vi "CAN.Cleanup.vi"(8 "error in (no error)":errorcluster, 11 "State Variables Out":T1={"Comm"=refnum, "Parameters"={"Name"="", "CAN"={"Interface"="", "Baud Rate"=0, "Diagnostic Protocol"=enum."GMLAN", "Transport Protocol"=enum."ISO TP - Normal Mode", "Transmit ID"=0, "Receive ID"=0, "Transmit Extension"=0, "Receive Extension"=0, "Receive UUDT ID"=0, "Enable Stream"=FALSE, "VW TP Channel ID"=0, "Fill Frame"=FALSE, "Fill Byte"=0, "Termination"=FALSE, "LIN Cluster"="", "NAD"=0, "IO Mode"=0, "Max DLC"=0, "FD Baud Rate"=0, "Timeout"=0, "FD ISO Mode"=0, "DoIP Address"="", "DoIP Source Address"=3584, "DoIP Dynamic Port"=TRUE, "DoIP Version"=2}, "986x"={"Enable"=FALSE, "RIO Device"="", "Bitfile"=path ""}, "Reads"=[], "Frames Lookup"=variant, "Writes"=[], "DPIDs"=[], "DPID Lookup"=variant, "DTC"={"Descriptor"={"DTC Byte Length"=0, "Status Byte Length"=0, "Add Data Byte Length"=0, "Byte Order"=enum."Motorola"}, "Value.Code"=[], "Value.String"=[], "Value.J2012String"=[], "Status.Code"=[], "Status.String"=[]}, "Created DTCs"=0, "Polls"=[], "Service Channels Status Lookup"=variant, "Trigger Lookup"=variant, "Security"={"Type"=enum."None", "Source DLL Path"=path "", "Target DLL Path"=path "", "Security Level"=0, "Static Master Key"="", "Max Key Length"=1, "Host IP Address"=""}, "Initial Comm State"=FALSE}, "ADCS Connection"={"Diag CAN Handle"=0, "Transport Protocol"=enum."ISO TP - Normal Mode", "Receive Address Extension"=0, "Transmit Address Extension"=0, "Receive CAN Id"=0, "Transmit CAN Id"=0, "Log Frames ?"=FALSE, "My TP Address"=0, "Other TP Address"=0, "T1"=0, "T2"=0, "T3"=0, "T4"=0, "Tx SN"=0, "Block Size"=0, "Rx SN"=0, "VW TP Initialized?"=FALSE, "Tx block no"=0, "baud rate"=0, "Interface"="", "Channel Diag CAN Handle"=0, "UDP Connection ID"=refnum, "TCP Connection ID"=refnum, "Target IP Addr"=0, "Source Address"=0, "Target Address"=0, "Send Header NACK?"=FALSE, "DLL Handle"=0, "NAD"=0, "Time Stamp read first"=0.0, "Time Stamp read last"=0.0, "Time Stamp write first"=0.0, "Time Stamp write last"=0.0, "Time Stamp write"=0.0, "Time Stamp read"=0.0, " I/O Mode"=0, "FD Baudrate"=0, "TX_DL"=0, "RX_DL"=0, "DoIP Protocol Version"=0, " Selected I/O Mode"=0, "TesterPresent Counter"=0, "TesterPresent Limit"=0, "TesterPresent Tick[ms]"=0, "TesterPresent RequireResponse?"=FALSE, "TesterPresent Stored Ref?"=FALSE, "TesterPresent Message"=[], "TesterPresent Task Handle"=0, "TesterPresent Semaphore"=refnum, "Response Plausibility Check"=0, "Default Version?"=FALSE, "Diagostic Globals"={"Timeout FC (Bs)"=0, "Timeout CF (Cr)"=0, "Timeout Diag Command"=0, "Receive Block Size (BS)"=0, "Wait Time CF (STmin)"=0, "Max Waits (N_WFTmax)"=0, "Waits to Send (N_WAIT)"=0, "Time between Waits (TW)"=0, "Fill CAN Frames?"=FALSE, "Fill Byte"=0, "Invalid Response as Error?"=FALSE, "Max RspPending Count"=0, "VWTP Command Timeout"=0, "Transport Protocol"=enum."ISO TP - Normal Mode", "Diag CAN Handle"=0, "DLL Handle"=0, "Timeout RspPending"=0}, "Session-based Properties?"=FALSE}, "XNET References"={"Database"="", "GMLAN.DPID.Frame"="", "Cluster.Convert"=""}, "XNETEngine (GMLAN)"=refnum, "Process"=refnum, "Reads"=refnum, "Writes"=refnum, "Cmds"=refnum, "DTCs"=refnum, "DTC Count"=refnum, "Status"=refnum, "Triggers"=refnum, "CANConnected"=refnum, "LocalStop"=refnum, "LocalCommStatus"=refnum, "Service Channels Status"=refnum, "Settings"=refnum, "Streaming Refs"={"Addon"="", "Port"="", "Filter Ref"=refnum, "Default Filter"={"ID Filters"=[], "Direction Filter"=enum."Tx/Rx", "Type Filter"=enum."All"}, "Port Settings"={"Mode"=0, "Baud Rate"=0, "Termination"=0, "FD ISO Mode"=0, "FD Baud Rate"=0}}} {"Streaming Refs"."Port Settings"."FD ISO Mode" items=["ISO", "Non ISO", "ISO Legacy"]; "Streaming Refs"."Port Settings"."Termination" items=["Off", "On"]; "Streaming Refs"."Port Settings"."Mode" items=["CAN 2.0", "CAN FD", "CAN FD+BRS"]; "ADCS Connection"."Diagostic Globals"."Fill Byte" format="%x"; "ADCS Connection"."TesterPresent Message" format="%.0x"; "ADCS Connection"."Selected I/O Mode" items=["CAN", "CAN FD", "CAN FD+BRS", "ECU Determined"]; "ADCS Connection"."DoIP Protocol Version" items=["2010"=1, "2012"=2]; "ADCS Connection"."RX_DL" items=["8"=8, "12"=12, "16"=16, "20"=20, "24"=24, "32"=32, "48"=48, "64"=64]; "ADCS Connection"."TX_DL" items=["8"=8, "12"=12, "16"=16, "20"=20, "24"=24, "32"=32, "48"=48, "64"=64]; "ADCS Connection"."I/O Mode" items=["CAN", "CAN FD", "CAN FD+BRS", "Not yet determined"]; "Parameters"."Writes"."Signals"."Byte Order" items=["Little Endian", "Big Endian"]; "Parameters"."Writes"."Signals"."Data Type" items=["Signed", "Unsigned", "IEEE Float"]; "Parameters"."CAN"."DoIP Version" items=["2010"=1, "2012"=2]; "Parameters"."CAN"."DoIP Source Address" format="%.0x"; "Parameters"."CAN"."FD ISO Mode" items=["ISO", "Non ISO", "ISO Legacy"]; "Parameters"."CAN"."IO Mode" items=["CAN 2.0", "CAN FD", "CAN FD+BRS"]; "Parameters"."CAN"."Fill Byte" format="%.0x"; "Parameters"."CAN"."VW TP Channel ID" format="%.0x"; "Parameters"."CAN"."Receive UUDT ID" format="%.0x"; "Parameters"."CAN"."Receive Extension" format="%.0x"; "Parameters"."CAN"."Transmit Extension" format="%.0x"; "Parameters"."CAN"."Receive ID" format="%.0x"; "Parameters"."CAN"."Transmit ID" format="%.0x"; "Parameters"."Reads"."Signals"."Byte Order" items=["Little Endian", "Big Endian"]; "Parameters"."Reads"."Signals"."Data Type" items=["Signed", "Unsigned", "IEEE Float"]}) -> (0 "error out":errorcluster)   [LabVIEW 2019, in "Diagnostics Addon Engine.lvlib"]
uses:
  Diagnostics Addon Engine.lvlib
  Types/Diagnostics.State.ctl
  <vilib>/NI/NI VeriStand Addon Network Comm/Engine/VeriStand Comm.lvclass
  <vilib>/NI/NIVS Inline Async API/_VS Inline Async API/Process/Process.lvclass
  Addon Shared/Types/SysDef.Compile.ctl
  Addon Shared/Types/CAN.ctl
  Addon Shared/Types/CAN.Interface.ctl
  Addon Shared/Types/Protocol.ctl
  Addon Shared/Types/Transport.ctl
  Addon Shared/Types/986x.ctl
  Addon Shared/Types/Frame.Compile.ctl
  Addon Shared/Types/Type.ctl
  Addon Shared/Types/Signal.ctl
  Addon Shared/Types/DPID.ctl
  Addon Shared/Types/DPID.Rate.ctl
  Addon Shared/Types/DTC.Settings.ctl
  Addon Shared/Types/DTC.Descriptor.ctl
  Addon Shared/Types/Poll.Compiled.ctl
  Addon Shared/Types/Security.ctl
  Addon Shared/Types/Security.Type.ctl
  <vilib>/Automotive Diagnostic Command Set/Diagnostic Transport.llb/Diag Reference.ctl
  <vilib>/Automotive Diagnostic Command Set/Diagnostic Transport.llb/Transport Protocol Selector.ctl
  <vilib>/Automotive Diagnostic Command Set/Diagnostic Transport.llb/DoIP Protocol Version.ctl
  <vilib>/Automotive Diagnostic Command Set/Diagnostic Transport.llb/Diag Globals.ctl
  Types/XNET.Refs.ctl
  <vilib>/NI/AMC/Message Queue.ctl
  <vilib>/NI/AMC/Message.ctl
  <vilib>/NI/Tools/Keyed Array/KeyedArray.ctl
  <vilib>/NI/NIVS Inline Async API/_Data Access Engine/Data Access Engine/Types/Write.DVR.ctl
  <vilib>/NI/NIVS Inline Async API/_Data Access Engine/Access Type Classes/Write/Write.lvclass
  <vilib>/NI/NIVS Inline Async API/_Data Access Engine/Data Access Engine/Types/Read.DVR.ctl
  <vilib>/NI/NIVS Inline Async API/_Data Access Engine/Access Type Classes/Read/Read.lvclass
  <vilib>/NI/NIVS Inline Async API/_Data Access Engine/Data Access Engine/Types/ReadWrite.DVR.ctl
  <vilib>/NI/NIVS Inline Async API/_Data Access Engine/Access Type Classes/ReadWrite/ReadWrite.lvclass
  SubModules/CAN-Streaming-Support/Source/Addon/Addon Engine/Types/Engine Stream Refs.ctl
  SubModules/CAN-Streaming-Support/Source/Addon/Addon Shared/Types/Direction Filter.ctl
  SubModules/CAN-Streaming-Support/Source/Addon/Addon Shared/Types/Type Filter.ctl
  SubModules/CAN-Streaming-Support/Source/Addon/Addon Shared/Types/Filter Parameters.ctl
  SubModules/CAN-Streaming-Support/Source/Addon/Addon Engine/Types/Engine Stream Port Settings.ctl
  <vilib>/NI/NIVS Inline Async API/_Data Access Engine/Access Type Classes/Write/Write.lvclass/Write.ctl
  <vilib>/NI/NIVS Inline Async API/_Data Access Engine/Data Access Engine/Methods/Write.Data.vi
  <vilib>/NI/NIVS Inline Async API/_Data Access Engine/Access Type Classes/Write/Write.ProcessData.vi
  <vilib>/NI/NIVS Inline Async API/_Data Access Engine/Access Type Classes/Write/Write.Buffer.vi
  <vilib>/NI/NIVS Inline Async API/_Data Access Engine/Access Type Classes/Write/Write.Commit.vi
  Addon Shared/SubVIs/Constants.vi
  <vilib>/xnet/xnet.llb/XNET Database Delete (Cluster).vi
  <vilib>/xnet/xnet.llb/XNET Database Close (Database).vi
  <vilib>/Utility/SystemLogging/Write to System Log.vi
  <vilib>/addons/Automotive Diagnostic Command Set/NI_Automotive Diagnostic Command Set.lvlib
  <vilib>/NI/NIVS Inline Async API/_Data Access Engine/Data Access Engine/Data Access Engine.lvclass
  Addon Shared/Diagnostics Addon Shared.lvlib
  <vilib>/NI/Tools/Keyed Array/Tools_KeyedArray.lvlib
  <vilib>/NI/AMC/AMC.lvlib
  SubModules/CAN-Streaming-Support/Source/Addon/Addon Engine/CAN Stream Support Engine.lvlib
  SubModules/CAN-Streaming-Support/Source/Addon/Addon Shared/CAN Stream Support Shared.lvlib
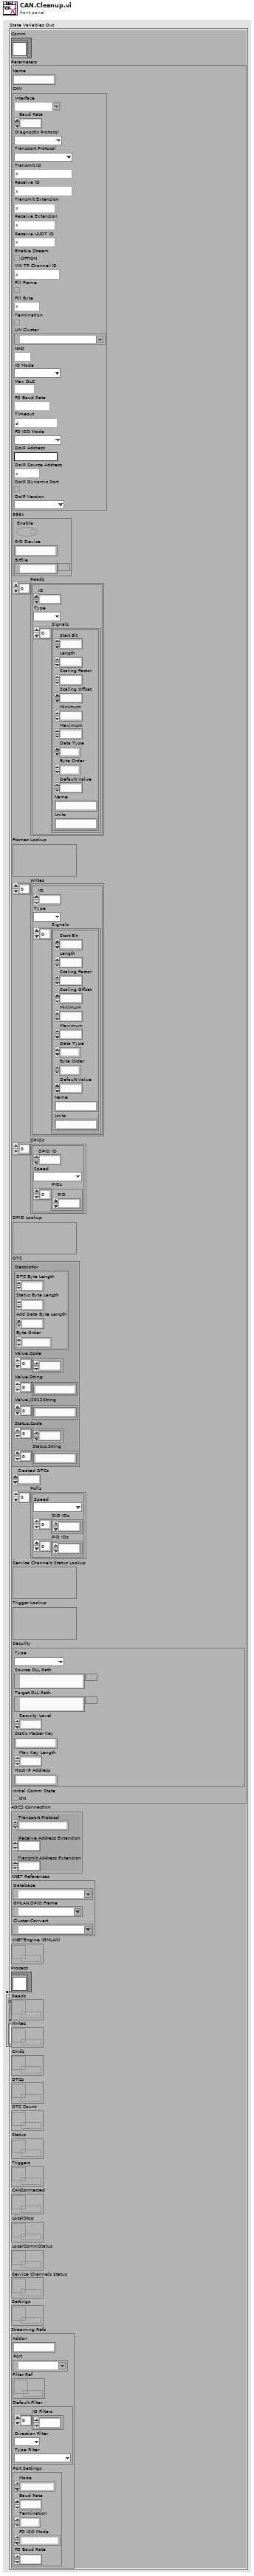
[diagram p1: front panel]
types:
  T1 = typedef "Diagnostics Addon Engine.lvlib/Diagnostics.State.ctl" = cluster{"Comm":refnum<class "VeriStand Comm.lvclass">, "Parameters":T2, "ADCS Connection":T18, "XNET References":T23, "XNETEngine (GMLAN)":T24, "Process":refnum<class "Process.lvclass">, "Reads":T25, "Writes":T26, "Cmds":T27, "DTCs":T25, "DTC Count":T25, "Status":T25, "Triggers":T27, "CANConnected":T25, "LocalStop":refnum<data-value>, "LocalCommStatus":refnum<data-value>, "Service Channels Status":T25, "Settings":T26, "Streaming Refs":T28}
  T2 = typedef "Diagnostics Addon Shared.lvlib/SysDef.Compile.ctl" = cluster{"Name":string, "CAN":T3, "986x":T7, "Reads":T8[], "Frames Lookup":variant, "Writes":T8[], "DPIDs":T11[], "DPID Lookup":variant, "DTC":T13, "Created DTCs":u32, "Polls":T15[], "Service Channels Status Lookup":variant, "Trigger Lookup":variant, "Security":T16, "Initial Comm State":bool}
  T3 = typedef "Diagnostics Addon Shared.lvlib/CAN.ctl" = cluster{"Interface":T4, "Baud Rate":u64, "Diagnostic Protocol":T5, "Transport Protocol":T6, "Transmit ID":u32, "Receive ID":u32, "Transmit Extension":u8, "Receive Extension":u8, "Receive UUDT ID":u32, "Enable Stream":bool, "VW TP Channel ID":u32, "Fill Frame":bool, "Fill Byte":u8, "Termination":bool, "LIN Cluster":refnum<k21>, "NAD":u8, "IO Mode":u32, "Max DLC":u16, "FD Baud Rate":u64, "Timeout":u32, "FD ISO Mode":u32, "DoIP Address":string, "DoIP Source Address":u16, "DoIP Dynamic Port":bool, "DoIP Version":u16}
  T4 = typedef "Diagnostics Addon Shared.lvlib/CAN.Interface.ctl" = string
  T5 = typedef "Diagnostics Addon Shared.lvlib/Protocol.ctl" = enum16{"GMLAN", "KWP-2000", "UDS", "User-Defined"}
  T6 = typedef "Diagnostics Addon Shared.lvlib/Transport.ctl" = enum16{"ISO TP - Normal Mode", "ISO TP - Mixed Mode", "VW TP 2.0", "Diagnostics on IP", "ISO TP LIN"}
  T7 = typedef "Diagnostics Addon Shared.lvlib/986x.ctl" = cluster{"Enable":bool, "RIO Device":string, "Bitfile":path}
  T8 = typedef "Diagnostics Addon Shared.lvlib/Frame.Compile.ctl" = cluster{"ID":u32, "Type":T9, "Signals":T10[]}
  T9 = typedef "Diagnostics Addon Shared.lvlib/Type.ctl" = enum16{"DID", "CDID", "PID", "CPID", "Read Memory", "Write Memory", "IO Control", "Routine Start", "Routine Request", "Routine Stop", "User Defined", "DTC Control", "Clear DTCs", "Read DTCs", "Start DTCs", "DTC Change Count", "Tester Present", "Unlock ECU", "Reset ECU", "Diag Session Control", "Communication Control", "DPID Control", "Poll Control", "Diag Comm Port Control"}
  T10 = typedef "Diagnostics Addon Shared.lvlib/Signal.ctl" = cluster{"Start Bit":u32, "Length":u32, "Scaling Factor":dbl, "Scaling Offset":dbl, "Minimum":dbl, "Maximum":dbl, "Data Type":u32, "Byte Order":u32, "Default Value":dbl, "Name":string, "Units":string}
  T11 = typedef "Diagnostics Addon Shared.lvlib/DPID.ctl" = cluster{"DPID ID":u8, "Speed":T12, "PIDs":u16[]}
  T12 = typedef "Diagnostics Addon Shared.lvlib/DPID.Rate.ctl" = enum16{"Slow", "Medium", "Fast"}
  T13 = typedef "Diagnostics Addon Shared.lvlib/DTC.Settings.ctl" = cluster{"Descriptor":T14, "Value.Code":dbl[], "Value.String":string[], "Value.J2012String":string[], "Status.Code":dbl[], "Status.String":string[]}
  T14 = typedef "Diagnostics Addon Shared.lvlib/DTC.Descriptor.ctl" = cluster{"DTC Byte Length":i32, "Status Byte Length":i32, "Add Data Byte Length":i32, "Byte Order":enum16{"Motorola", "Intel"}}
  T15 = typedef "Diagnostics Addon Shared.lvlib/Poll.Compiled.ctl" = cluster{"Speed":T12, "DID IDs":u32[], "PID IDs":u32[]}
  T16 = typedef "Diagnostics Addon Shared.lvlib/Security.ctl" = cluster{"Type":T17, "Source DLL Path":path, "Target DLL Path":path, "Security Level":u8, "Static Master Key":string, "Max Key Length":u32, "Host IP Address":string}
  T17 = typedef "Diagnostics Addon Shared.lvlib/Security.Type.ctl" = enum16{"None", "SeedKey DLL", "MasterKey (Channel)", "MasterKey (Static)", "SeedKey DLL (Windows)"}
  T18 = typedef "NI_Automotive Diagnostic Command Set.lvlib/Diag Reference.ctl" = cluster{"Diag CAN Handle":u32, "Transport Protocol":T19, "Receive Address Extension":u8, "Transmit Address Extension":u8, "Receive CAN Id":u32, "Transmit CAN Id":u32, "Log Frames ?":bool, "My TP Address":u8, "Other TP Address":u8, "T1":u16, "T2":u16, "T3":u16, "T4":u16, "Tx SN":u8, "Block Size":u8, "Rx SN":u8, "VW TP Initialized?":bool, "Tx block no":u8, "baud rate":u64, "Interface":string, "Channel Diag CAN Handle":u32, "UDP Connection ID":refnum<k16>, "TCP Connection ID":refnum<k5>, "Target IP Addr":u32, "Source Address":u16, "Target Address":u16, "Send Header NACK?":bool, "DLL Handle":u32, "NAD":u8, "Time Stamp read first":dbl, "Time Stamp read last":dbl, "Time Stamp write first":dbl, "Time Stamp write last":dbl, "Time Stamp write":dbl, "Time Stamp read":dbl, " I/O Mode":u32, "FD Baudrate":u64, "TX_DL":u16, "RX_DL":u16, "DoIP Protocol Version":T20, " Selected I/O Mode":u32, "TesterPresent Counter":u32, "TesterPresent Limit":u32, "TesterPresent Tick[ms]":i32, "TesterPresent RequireResponse?":bool, "TesterPresent Stored Ref?":bool, "TesterPresent Message":u8[], "TesterPresent Task Handle":i32, "TesterPresent Semaphore":T21, "Response Plausibility Check":u32, "Default Version?":bool, "Diagostic Globals":T22, "Session-based Properties?":bool}
  T19 = typedef "NI_Automotive Diagnostic Command Set.lvlib/Transport Protocol Selector.ctl" = enum16{"ISO TP - Normal Mode", "ISO TP - Mixed Mode", "VW TP 2.0", "Diagnostics on IP", "ISO TP LIN"}
  T20 = typedef "NI_Automotive Diagnostic Command Set.lvlib/DoIP Protocol Version.ctl" = u8
  T21 = typedef "Semaphore RefNum" = refnum<k1>
  T22 = typedef "NI_Automotive Diagnostic Command Set.lvlib/Diag Globals.ctl" = cluster{"Timeout FC (Bs)":u32, "Timeout CF (Cr)":u32, "Timeout Diag Command":u32, "Receive Block Size (BS)":u8, "Wait Time CF (STmin)":u8, "Max Waits (N_WFTmax)":u8, "Waits to Send (N_WAIT)":i32, "Time between Waits (TW)":u32, "Fill CAN Frames?":bool, "Fill Byte":u32, "Invalid Response as Error?":bool, "Max RspPending Count":u32, "VWTP Command Timeout":u32, "Transport Protocol":T19, "Diag CAN Handle":u32, "DLL Handle":u32, "Timeout RspPending":u32}
  T23 = typedef "Diagnostics Addon Engine.lvlib/XNET.Refs.ctl" = cluster{"Database":refnum<k21>, "GMLAN.DPID.Frame":refnum<k21>, "Cluster.Convert":refnum<k21>}
  T24 = typedef "AMC.lvlib/Message Queue.ctl" = refnum<queue>
  T25 = typedef "Data Access Engine.lvlib/Data Access Engine.lvclass/Write.DVR.ctl" = refnum<data-value>
  T26 = typedef "Data Access Engine.lvlib/Data Access Engine.lvclass/Read.DVR.ctl" = refnum<data-value>
  T27 = typedef "Data Access Engine.lvlib/Data Access Engine.lvclass/ReadWrite.DVR.ctl" = refnum<data-value>
  T28 = typedef "CAN Stream Support Engine.lvlib/Engine Stream Refs.ctl" = cluster{"Addon":string, "Port":refnum<k21>, "Filter Ref":refnum<data-value>, "Default Filter":T29, "Port Settings":T32}
  T29 = typedef "CAN Stream Support Shared.lvlib/Filter Parameters.ctl" = cluster{"ID Filters":u32[], "Direction Filter":T30, "Type Filter":T31}
  T30 = typedef "CAN Stream Support Shared.lvlib/Direction Filter.ctl" = enum16{"Tx/Rx", "Rx", "Tx"}
  T31 = typedef "CAN Stream Support Shared.lvlib/Type Filter.ctl" = enum16{"All", "CAN Data", "CAN Remote", "CAN Bus Error", "CAN 2.0 Data", "CAN FD Data", "CAN FD+BRS Data", "J1939 Data", "Delay", "Log Trigger", "Start Trigger"}
  T32 = typedef "CAN Stream Support Engine.lvlib/Engine Stream Port Settings.ctl" = cluster{"Mode":u32, "Baud Rate":u64, "Termination":u32, "FD ISO Mode":u32, "FD Baud Rate":u64}
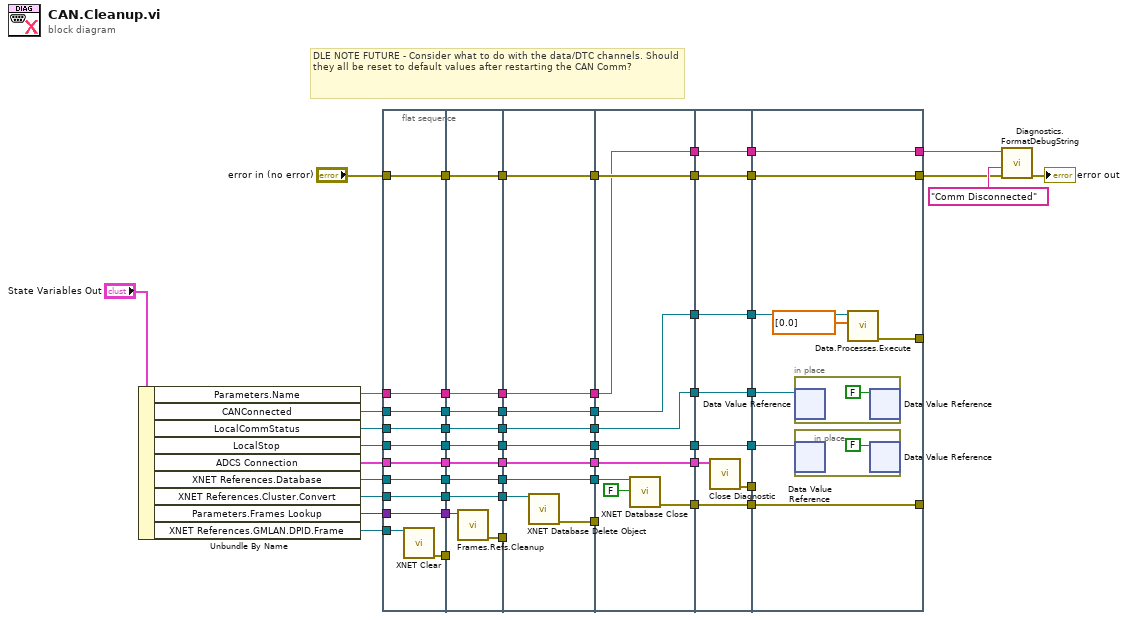
[diagram p0: block diagram]
diagram:
  # "DLE NOTE FUTURE - Consider what to do with the data/DTC channels. Should they all be reset to default values after restarting the CAN Comm?"
  n1 = Unbundle By Name("State Variables Out") -> ("Parameters.Name"=w13:string, "CANConnected"=w26:T25, "LocalCommStatus"=w27:refnum<data-value>, "LocalStop"=w25:refnum<data-value>, "ADCS Connection"=w22:T18, "XNET References.Database"=w21:refnum<k21>, "XNET References.Cluster.Convert"=w20:refnum<k21>, "Parameters.Frames Lookup"=w19:variant, "XNET References.GMLAN.DPID.Frame"=w18:refnum<k21>)
  n2 = flat-sequence {
    tunnel: w20 -> [w66]
    tunnel: w19 -> [w67]
    tunnel: [w67] -> w56
    tunnel: [w66] -> w55
    tunnel: w18 -> [w65]
    tunnel: [w64] -> w54
    tunnel: [w63] -> w53
    tunnel: w22 -> [w63]
    tunnel: [w62] -> w52
    tunnel: w21 -> [w62]
    tunnel: "error in (no error)" -> [w61]
    tunnel: [w61] -> w51
    tunnel: [w60] -> w50
    tunnel: w25 -> [w60]
    tunnel: [w59] -> w49
    tunnel: w26 -> [w59]
    tunnel: w27 -> [w58]
    tunnel: [w58] -> w48
    tunnel: [w57] -> w14
    tunnel: w13 -> [w57]
    tunnel: [w77] -> w47
    tunnel: w56 -> [w76]
    tunnel: w55 -> [w77]
    tunnel: w54 -> [_]
    tunnel: [w75] -> w46
    tunnel: w53 -> [w75]
    tunnel: [w74] -> w45
    tunnel: w52 -> [w74]
    tunnel: [w73] -> w44
    tunnel: [w72] -> w43
    tunnel: w51 -> [w72]
    tunnel: [w71] -> w42
    tunnel: w50 -> [w71]
    tunnel: [w70] -> w41
    tunnel: w49 -> [w70]
    tunnel: [w69] -> w40
    tunnel: w48 -> [w69]
    tunnel: [w68] -> w15
    tunnel: w14 -> [w68]
    tunnel: [w86] -> w8
    tunnel: [w85] -> w7
    tunnel: [w84] -> w6
    tunnel: [w83] -> w5
    tunnel: [w82] -> w4
    tunnel: [w81] -> w3
    tunnel: [w80] -> w2
    tunnel: w15 -> [w80]
    tunnel: w40 -> [w81]
    tunnel: w41 -> [w82]
    tunnel: w42 -> [w83]
    tunnel: w43 -> [w84]
    tunnel: w44 -> [_]
    tunnel: w45 -> [w85]
    tunnel: w46 -> [w86]
    tunnel: w47 -> [w79]
    tunnel: [w78] -> w1
    tunnel: [w93] -> w39
    tunnel: w8 -> [w95]
    tunnel: [w95] -> w38
    tunnel: w7 -> [w94]
    tunnel: [w91] -> w37
    tunnel: w6 -> [w91]
    tunnel: [w90] -> w36
    tunnel: w5 -> [w90]
    tunnel: [w89] -> w35
    tunnel: w4 -> [w89]
    tunnel: [w88] -> w34
    tunnel: w3 -> [w88]
    tunnel: [w87] -> w16
    tunnel: w2 -> [w87]
    tunnel: w1 -> [_]
    tunnel: w39 -> [w103]
    tunnel: w38 -> [w102]
    tunnel: w37 -> [w101]
    tunnel: [w103] -> w33
    tunnel: [w101] -> w32
    tunnel: [w100] -> w31
    tunnel: [w99] -> w30
    tunnel: w36 -> [w99]
    tunnel: w35 -> [w98]
    tunnel: [w98] -> w29
    tunnel: [w97] -> w28
    tunnel: w34 -> [w97]
    tunnel: [w96] -> w17
    tunnel: w16 -> [w96]
    tunnel: [w110] -> w10
    tunnel: [w111] -> _
    tunnel: w33 -> [w111]
    tunnel: w32 -> [w110]
    tunnel: w31 -> [_]
    tunnel: w30 -> [w109]
    tunnel: w29 -> [w107]
    tunnel: [w106] -> _
    tunnel: w28 -> [w105]
    tunnel: w17 -> [w104]
    tunnel: [w104] -> w11
    frame #0 {
      n3 = call <vilib>:"XNET Clear.vi"("session in"=w65) -> ("error out"=w64:errorcluster)  [unwired: 14 in]
    }
    frame #1 {
      n4 = call "Frames.Refs.Cleanup.vi"("Lookup"=w76) -> ("Array"=w73:errorcluster[])  [unwired: 10 in]
    }
    frame #2 {
      n5 = call-poly <vilib>:"XNET Database Delete Object.vi"("cluster in"=w79) -> ("error out"=w78:errorcluster)  [unwired: 14 in]
    }
    frame #3 {
      n6 = call-poly <vilib>:"XNET Database Close.vi"("database in"=w94, "close all? (true)"=FALSE) -> ("error out"=w93:errorcluster)  [unwired: 13 in]
    }
    frame #4 {
      n7 = call <vilib>:"Close Diagnostic.vi"("diag ref in"=w102) -> ("error out"=w100:errorcluster)  [unwired: 10 in]
    }
    frame #5 {
      n8 = in-place {
        n9 = in-place-dvr #1(w105) -> ()  [unwired: 2 out]
        n10 = in-place-dvr #1(FALSE ("data value")) -> ()  [unwired: 2 out]
      }
      n11 = in-place {
        n12 = in-place-dvr #2(w109) -> ()  [unwired: 2 out]
        n13 = in-place-dvr #2(FALSE ("data value")) -> ()  [unwired: 2 out]
      }
      n14 = call-poly <vilib>:"Data.Processes.Execute.vi"("Values"=dbl[] [0.0], "Ref"=w107) -> ("error out"=w106:errorcluster)  [unwired: 9 in]
    }
  }
  n15 = call "Diagnostics.FormatDebugString.vi"("error in (no error)"=w10, "State"="Comm Disconnected" ("Message"), "Name"=w11) -> ("error out"=→"error out":errorcluster)  [unwired: 8 in]
